vi "HapticSTM2.vi"() -> ()   [LabVIEW 2017]
uses:
  <userlib>/PositionDLL/PositionDLL.lvlib
panel:
  out "Origin Y":dbl
  out "Origin X":dbl
  out "Arm output":dbl
  in  "Rough adjust":dbl
  out "ZVAL":dbl
  out "Y Out":dbl
  out "X Out":dbl
  out "Max speed":dbl
  out "Width":dbl
  out "VY":dbl
  out "VZ":dbl
  out "VX":dbl
  in  "Drag":dbl=1.0
  in  "STOP":bool
  in  "START":bool
  out "Fy":dbl
  out "Fz":dbl
  out "phi":dbl
  out "psi":dbl
  out "Fx":dbl
  out "theta":dbl
  out "x":dbl
  out "y":dbl
  out "z":dbl
  in  "Fine adjust":dbl=3.5
  out "Clicks":dbl
  out "Height":dbl
  # "Sample Window"
  # "Position"
  # "Sensitivity"
  # "Force"
  # "STM I/O"
  # "Angles"
  # "Velocity"
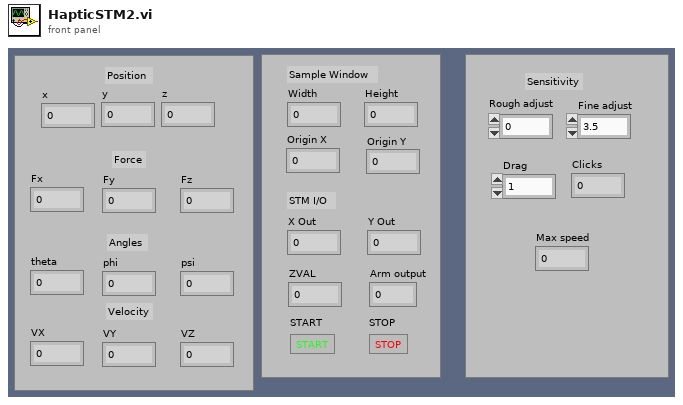
[diagram p1: front panel]
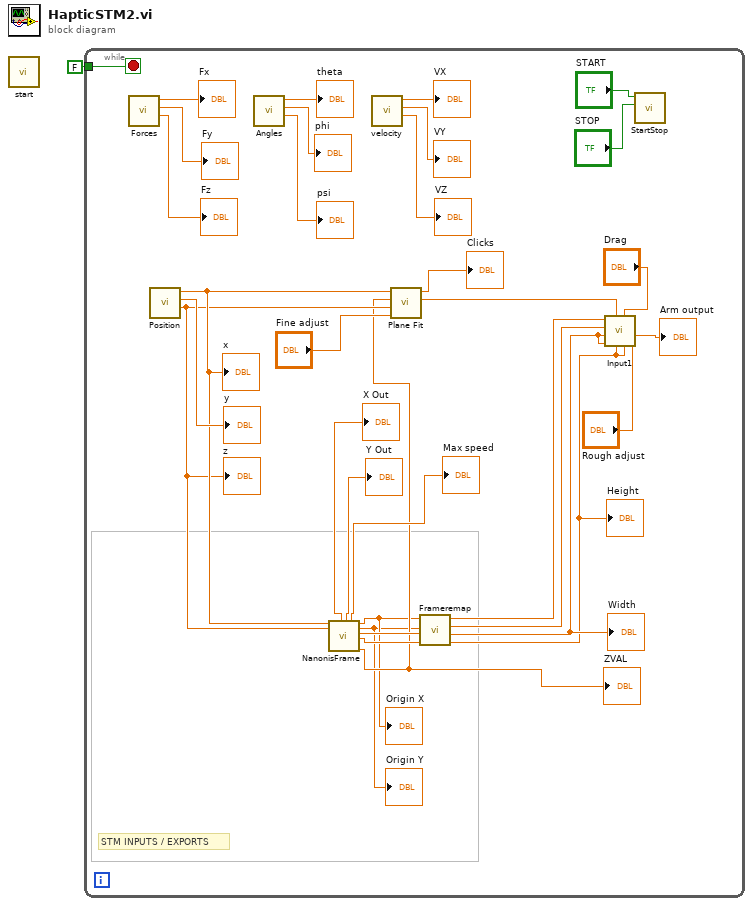
[diagram p0: block diagram]
diagram:
  n1 = call <userlib>:"start.vi"() -> ()  [unwired: 11 in, 1 out]
  n2 = while {
    tunnel: FALSE -> [w22]
    stop <- w22 stop-if-true
    # "STM INPUTS / EXPORTS"
    n3 = call <userlib>:"Forces.vi"() -> ("Fz"=→"Fz":dbl, "Fy"=→"Fy":dbl, "Fx"=→"Fx":dbl)  [unwired: 9 in]
    n4 = call <userlib>:"Position.vi"() -> ("Z"=w12:dbl, "Y"=→"y":dbl, "X"=w13:dbl)  [unwired: 9 in]
    "x" <- w13
    "z" <- w12
    n5 = call <userlib>:"Angles.vi"() -> ("psi"=→"psi":dbl, "phi"=→"phi":dbl, "theta"=→"theta":dbl)  [unwired: 9 in]
    n6 = call <userlib>:"NanonisFrame.vi"("x"=w13, "z"=w12) -> ("X Out"=→"X Out":dbl, "Z Out"=→"Y Out":dbl, "Speed"=→"Max speed":dbl, "FO X"=w3:dbl, "FO Z"=w2:dbl, "FW"=w8:dbl, "FH"=w7:dbl, "CVAL (nA)"=w4:dbl)  [unwired: 10 in]
    "ZVAL" <- w4
    "Origin X" <- w3
    "Origin Y" <- w2
    n7 = call <userlib>:"velocity.vi"() -> ("VZ"=→"VZ":dbl, "VY"=→"VY":dbl, "VX"=→"VX":dbl)  [unwired: 9 in]
    n8 = call <userlib>:"Plane Fit.vi"("Sensitivity"="Fine adjust", "Z"=w12, "Nano Z"=w4, "X"=w13) -> ("Output"=w26:dbl, "Clicks"=→"Clicks":dbl)  [unwired: 6 in]
    n9 = call <userlib>:"Frameremap.vi"("FH"=w7, "FW"=w8, "FO Z"=w2, "FO X"=w3) -> ("FH"=w14:dbl, "FW"=w15:dbl, "Z Origin"=w24:dbl, "X Origin"=w25:dbl)  [unwired: 4 in]
    "Height" <- w14
    "Width" <- w15
    n10 = call <userlib>:"Input1.vi"("Current * 10^input"="Rough adjust", "Scopez"=w14, "Drag"="Drag", "FH"=w14, "Signal in"=w26, "FW"=w15, "Scopex"=w15, "Z origin"=w24, "X origin"=w25) -> ("Scaled Current"=→"Arm output":dbl)  [unwired: 2 in]
    n11 = call <userlib>:"StartStop.vi"("STOP"="STOP", "START"="START") -> ()  [unwired: 10 in]
  }
